vi "AlliGator Get Python Plugin Functions List.vi"(8 "Error In":errorcluster, 9 "Include Example Plugins":bool, 11 "Python Plugins Folder Path":path) -> (0 "Error Out":errorcluster, 3 "Array of Python Functions":T1[](array[typedef]))   [LabVIEW 2021, in "AlliGator Python Plugins.lvlib"]
doc: "Extracts list of python plugin functions from the Python Plugin folder."
uses:
  AlliGator Python Plugins.lvlib
  AlliGator Python Function Information.ctl
  AlliGator Python Function Parameter Definition.ctl
  AlliGator Python Function Output Definition.ctl
  AlliGator Python Plugin Target Type.ctl
panel:
  # "see the AlliGator License on the block diagram (Ctrl+E or Window:Show Block Diagram)"
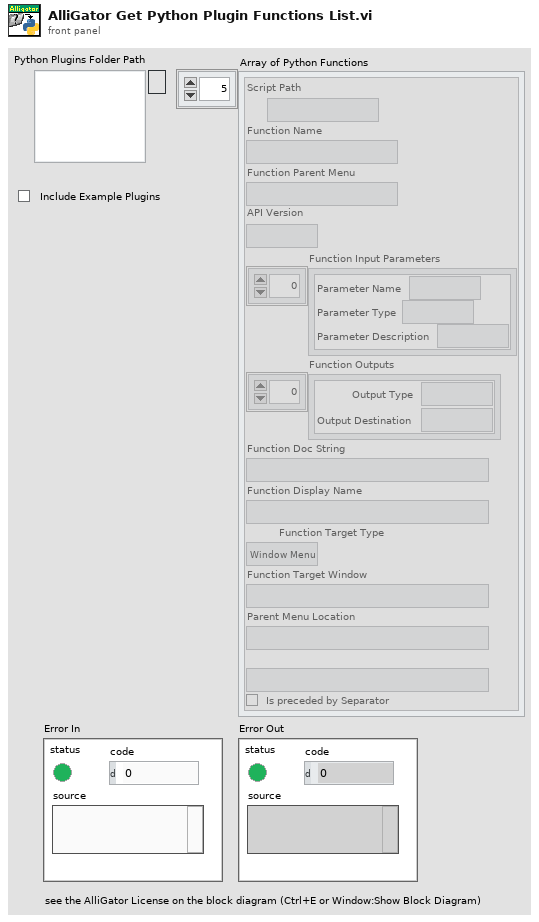
[diagram p1: front panel]
types:
  T1 = typedef "AlliGator Python Plugins.lvlib/AlliGator Python Function Information.ctl" = cluster{"Script Path":path, "Function Name":string, "Function Parent Menu":string, "API Version":string, "Function Input Parameters":T2[], "Function Outputs":T3[], "Function Doc String":string, "Function Display Name":string, "Function Target Type":T4, "Function Target Window":string, "Parent Menu Location":string, "Item Menu Tag":string, "Is preceded by Separator":bool}
  T2 = typedef "AlliGator Python Plugins.lvlib/AlliGator Python Function Parameter Definition.ctl" = cluster{"Parameter Name":string, "Parameter Type":string, "Parameter Description":string}
  T3 = typedef "AlliGator Python Plugins.lvlib/AlliGator Python Function Output Definition.ctl" = cluster{"Output Type":string, "Output Destination":string}
  T4 = typedef "AlliGator Python Plugins.lvlib/AlliGator Python Plugin Target Type.ctl" = enum16{"Undefined", "Window Menu", "Object Menu"}
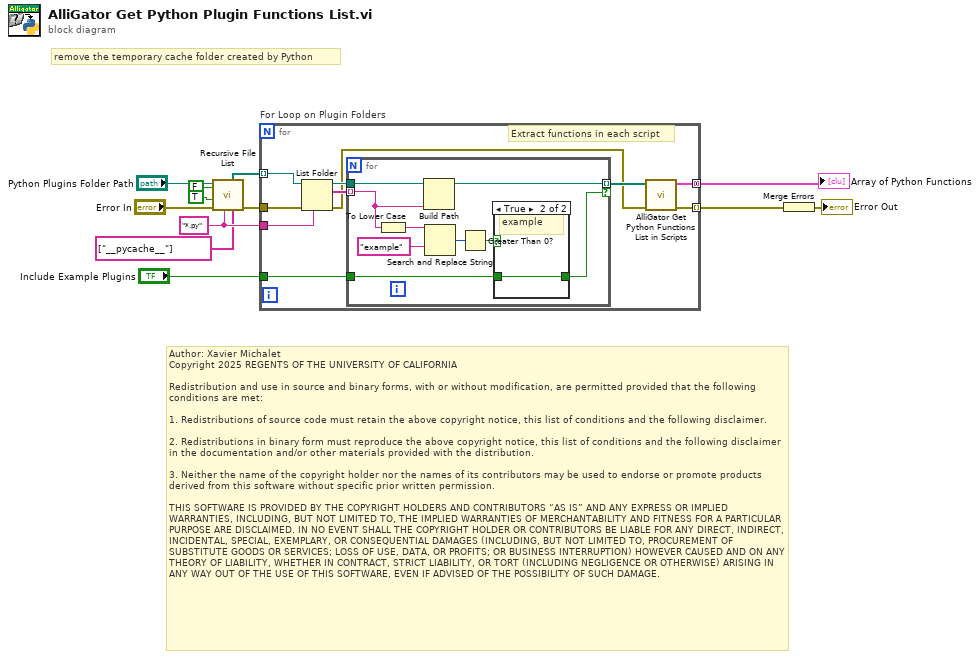
[diagram p0: block diagram]
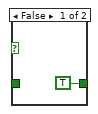
[diagram p2: hidden frame]
diagram:
  w7 = "*.py" ("pattern")
  # "Author: Xavier Michalet\nCopyright 2025 REGENTS OF THE UNIVERSITY OF CALIFORNIA\n\nRedistribution and use in source and binary forms, with or without modification, are permitted provided that the following conditions are met:\n\n1. Redistributions of source code must retain the above copyright notice, this list of conditions and the following disclaimer.\n\n2. Redistributions in binary form must reproduce the above copyright notice, this list of conditions and the following disclaimer in the documentation and/or other materials provided with the distribution.\n\n3. Neither the name of the copyright holder nor the names of its contributors may be used to endorse or promote products derived from this software without specific prior written permission.\n\nTHIS SOFTWARE IS PROVIDED BY THE COPYRIGHT HOLDERS AND CONTRIBUTORS “AS IS” AND ANY EXPRESS OR IMPLIED WARRANTIES, INCLUDING, BUT NOT LIMITED TO, THE IMPLIED WARRANTIES OF MERCHANTABILITY AND FITNESS FOR A PARTICULAR PURPOSE ARE DISCLAIMED. IN NO EVENT SHALL THE COPYRIGHT HOLDER OR CONTRIBUTORS BE LIABLE FOR ANY DIRECT, INDIRECT, INCIDENTAL, SPECIAL, EXEMPLARY, OR CONSEQUENTIAL DAMAGES (INCLUDING, BUT NOT LIMITED TO, PROCUREMENT OF SUBSTITUTE GOODS OR SERVICES; LOSS OF USE, DATA, OR PROFITS; OR BUSINESS INTERRUPTION) HOWEVER CAUSED AND ON ANY THEORY OF LIABILITY, WHETHER IN CONTRACT, STRICT LIABILITY, OR TORT (INCLUDING NEGLIGENCE OR OTHERWISE) ARISING IN ANY WAY OUT OF THE USE OF THIS SOFTWARE, EVEN IF ADVISED OF THE POSSIBILITY OF SUCH DAMAGE."
  # "remove the temporary cache folder created by Python"
  n1 = call <vilib>:"Recursive File List.vi"("Folders to Exclude"=string[] ["__pycache__"], "pattern"=w7, "error in (no error)"="Error In", "Continue Recursing on Error? (F)"=TRUE, "Treat LLBs as Folders?"=FALSE, "Folder Path"="Python Plugins Folder Path") -> ("error out"=w8:errorcluster, "All Folders"=w4:path[])  [unwired: 1 in, 3 out]
  n2 = for "For Loop on Plugin Folders" {
    tunnel: w4 -> [w22] mode=indexing
    tunnel: w7 -> [w20]
    tunnel: [w17] -> w3 mode=concatenating
    tunnel: w8 -> [w21]
    tunnel: [w18] -> w6 mode=indexing
    tunnel: "Include Example Plugins" -> [w16]
    # "Extract functions in each script"
    n3 = List Folder(path=w22, pattern=w20, error in=w21) -> (path out=w15:path, filenames=w14:string[], error out=w13:errorcluster)  [unwired: 1 in, 1 out]
    n4 = for {
      tunnel: w15 -> [w31]
      tunnel: w14 -> [w29] mode=indexing
      tunnel: [w30] -> w19 mode=indexing if=w23
      tunnel: w16 -> [w24]
      n5 = To Lower Case(string=w29) -> (all lower case string=w27:string)
      n6 = Build Path(base path=w31, name or relative path=w29) -> (appended path=w30:path)
      n7 = Search and Replace String(input string=w27, search string="example") -> (number of replacements=w26:i32)  [unwired: 6 in, 3 out]
      n8 = Greater Than 0?(x=w26) -> (x > 0?=w25:bool)
      n9 = case shown="True" w25 {
        tunnel: w24 -> [_ w33]
        tunnel: [TRUE ("Include Example Plugins") w33] -> w23
        frame False {
        }
        frame True {
          # "example"
        }
      }
    }
    n10 = call "AlliGator Get Python Functions List in Scripts.vi"("error in (no error)"=w13, "All Files in Dir"=w19) -> ("error out"=w18:errorcluster, "Array of Python Functions"=w17:T1[])  [unwired: 7 in, 1 out]
  }
  "Array of Python Functions" <- w3
  n11 = Merge Errors(w6) -> (→"Error Out":errorcluster)
